vi "Verify if Reports folder exist (SubVI).vi"(8 "error in (no error)":errorcluster, 9 "שם הממסר":string, 10 "File Type":string=".doc", 11 "Folder Name":string) -> (0 "error out":errorcluster, 3 "Path":path)   [LabVIEW 2014]
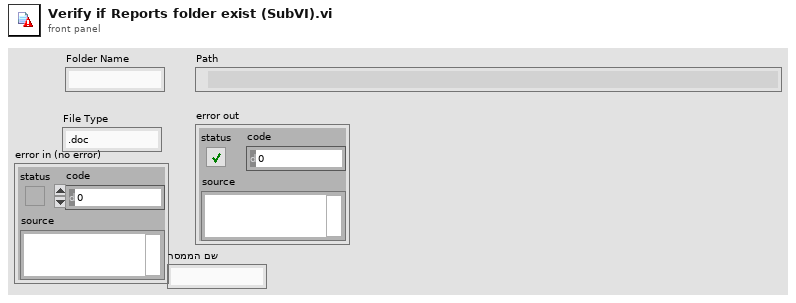
[diagram p1: front panel]
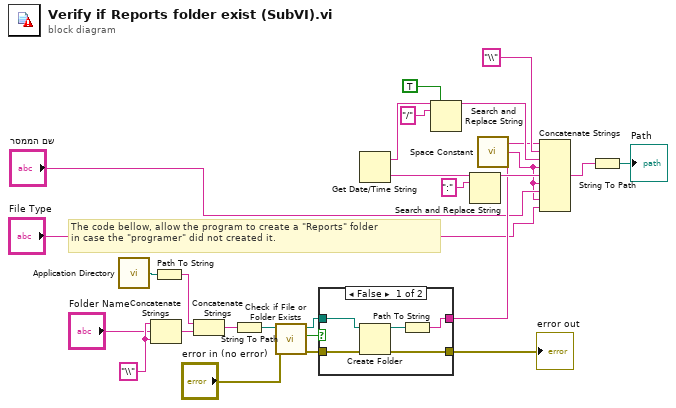
[diagram p0: block diagram]
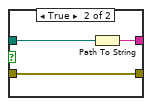
[diagram p2: hidden frame]
diagram:
  w7 = "\\" ("string")
  # "The code bellow, allow the program to create a \"Reports\" folder\nin case the \"programer\" did not created it."
  n1 = call <vilib>:"Application Directory.vi"() -> ("Application Directory"=w15:path)
  n2 = Concatenate Strings(w7, "Folder Name", w7) -> (w5:string)
  n3 = Path To String(path=w15) -> (string=w14:string)
  n4 = Concatenate Strings(w14, w5) -> (w16:string)
  n5 = String To Path(string=w16) -> (path=w13:path)
  n6 = call <vilib>:"Check if File or Folder Exists.vi"("error in (no error)"="error in (no error)", "path"=w13) -> ("error out"=w10:errorcluster, "file or folder exists?"=w12:bool, "dup path"=w11:path)  [unwired: 7 in]
  n7 = case shown="False" w12 {
    tunnel: w11 -> [w31 w34]
    tunnel: w10 -> [w30 w32]
    tunnel: [w28 w33] -> w9
    tunnel: [w27 w32] -> w8
    frame False {
      n8 = Create Folder(path (use dialog)=w31, error in=w30) -> (created path=w29:path, error out=w27:errorcluster)  [unwired: 1 in, 1 out]
      n9 = Path To String(path=w29) -> (string=w28:string)
    }
    frame True {
      n10 = Path To String(path=w34) -> (string=w33:string)
    }
  }
  "error out" <- w8
  n11 = Get Date/Time String() -> (date string=w22:string, time string=w25:string)  [unwired: 3 in]
  n12 = Search and Replace String(replace all?=TRUE, input string=w22, search string="/") -> (result string=w20:string)  [unwired: 5 in, 3 out]
  n13 = Search and Replace String(input string=w25, search string=":") -> (result string=w18:string)  [unwired: 6 in, 3 out]
  n14 = call <vilib>:"Space Constant.vi"() -> ("String"=w1:string)
  n15 = Concatenate Strings(w9, "\\" ("string"), w20, w1, w18, w1, "שם הממסר", w1, "File Type") -> (w19:string)
  n16 = String To Path(string=w19) -> (path=→"Path":path)
